vi "温度计 (子VI).vi"(10 "温度下限":dbl=10.0, 11 "温度上限":dbl=50.0) -> (1 "状态显示":string, 2 "温度计":dbl(slide) scale=0.0..100.0, 3 "报警显示":bool)   [LabVIEW 2025]
panel:
  in  "停止":bool
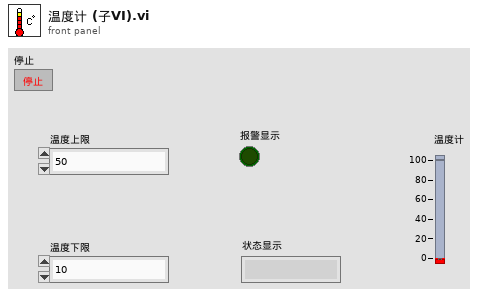
[diagram p1: front panel]
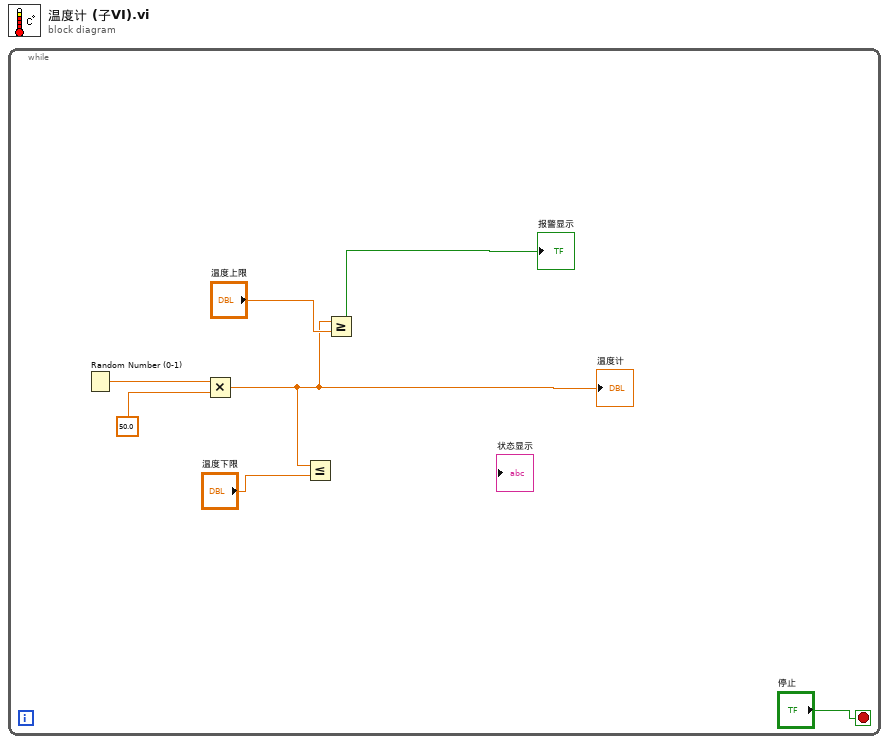
[diagram p0: block diagram]
diagram:
  n1 = while {
    stop <- "停止" stop-if-true
    n2 = Random Number (0-1)() -> (number: 0 to 1=w7:dbl)
    n3 = Multiply(x=w7, y=50.0) -> (x*y=w2:dbl)
    "温度计" <- w2
    n4 = Less Or Equal?(x=w2, y="温度下限") -> ()  [unwired: 1 out]
    n5 = Greater Or Equal?(x=w2, y="温度上限") -> (x >= y?=→"报警显示":bool)
  }
